vi "Read_Logitech.vi"() -> ()   [LabVIEW 2018]
uses:
  <vilib>/Utility/inputDevices.llb/joystickAcquire.vi
  <vilib>/Utility/inputDevices.llb/closeJoystick.vi
panel:
  out "X velocity":dbl
  out "Y velocity":dbl
  out "Angular Velocity":dbl
  out "axis info":T1
  out "error out":errorcluster
  out "direction info 2":T2={"pov 1"=-1, "pov 2"=-1, "pov 3"=-1, "pov 4"=-1}
  in  "stop":bool
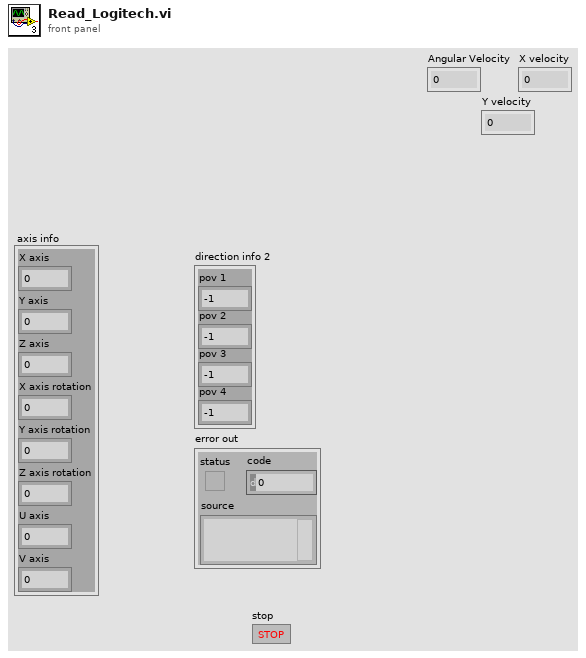
[diagram p1: front panel]
types:
  T1 = cluster{"X axis":i32, "Y axis":i32, "Z axis":i32, "X axis rotation":i32, "Y axis rotation":i32, "Z axis rotation":i32, "U axis":i32, "V axis":i32}
  T2 = cluster{"pov 1":i32, "pov 2":i32, "pov 3":i32, "pov 4":i32}
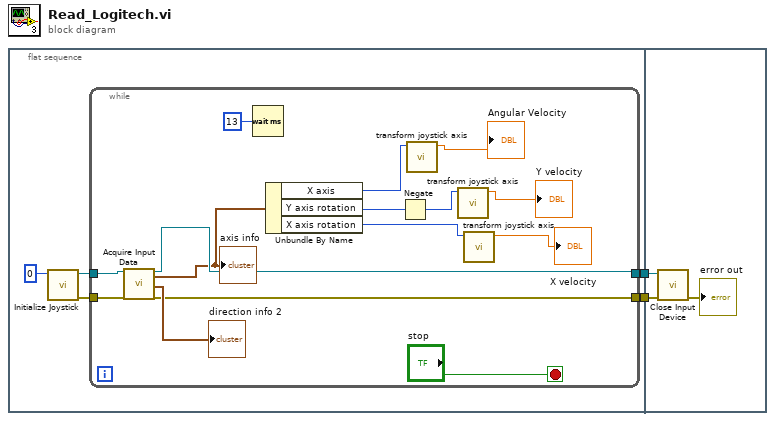
[diagram p0: block diagram]
diagram:
  n1 = flat-sequence {
    tunnel: [w5] -> w2
    tunnel: [w4] -> w1
    tunnel: w2 -> [w25]
    tunnel: w1 -> [w24]
    frame #0 {
      n2 = call <vilib>:"Initialize Joystick.vi"("device index"=0) -> ("error out"=w6:errorcluster, "device ID"=w7:refnum<k1>)  [unwired: 9 in]
      n3 = while {
        tunnel: w7 -> [w21]
        tunnel: w6 -> [w20]
        tunnel: [w19] -> w5
        tunnel: [w17] -> w4
        stop <- "stop" stop-if-true
        n4 = call-poly <vilib>:"Acquire Input Data.vi"("device ID"=w21, "error in (no error)"=w20) -> ("device ID"=w19:refnum<k1>, "axis info"=w15:T1, "direction info"=→"direction info 2":T2, "error out"=w17:errorcluster)  [unwired: 13 in, 1 out]
        "axis info" <- w15
        n5 = Wait (ms)(milliseconds to wait=u32 13) -> ()  [unwired: 1 out]
        n6 = Unbundle By Name(w15) -> ("X axis"=w13:i32, "Y axis rotation"=w14:i32, "X axis rotation"=w9:i32)
        n7 = Negate(x=w14) -> (-x=w11:i32)
        n8 = call <vilib>:"transform joystick axis.vi"("Axis Input"=w13) -> ("Output (-1..1)"=→"Angular Velocity":dbl)  [unwired: 10 in]
        n9 = call <vilib>:"transform joystick axis.vi"("Axis Input"=w11) -> ("Output (-1..1)"=→"Y velocity":dbl)  [unwired: 10 in]
        n10 = call <vilib>:"transform joystick axis.vi"("Axis Input"=w9) -> ("Output (-1..1)"=→"X velocity":dbl)  [unwired: 10 in]
      }
    }
    frame #1 {
      n11 = call-poly <vilib>:"Close Input Device.vi"("error in (no error)"=w24, "device ID"=w25) -> ("error out"=→"error out":errorcluster)  [unwired: 8 in]
    }
  }
